vi "Utils - Convert1Dto2DImage.vi"(8 "error in (no error)":errorcluster, 9 "1DImageData In":u8[](array[numeric])) -> (0 "error out":errorcluster, 1 "1DImageData Out":u8[](array[numeric]), 2 "ImageData2D":u8[][](array[numeric]))   [LabVIEW 2015]
doc: "Convert 1d U8 Image array to LabVIEW image. This VI supports only Mono8 image format."
uses:
  xiImageManager/xiImageMng - State.ctl
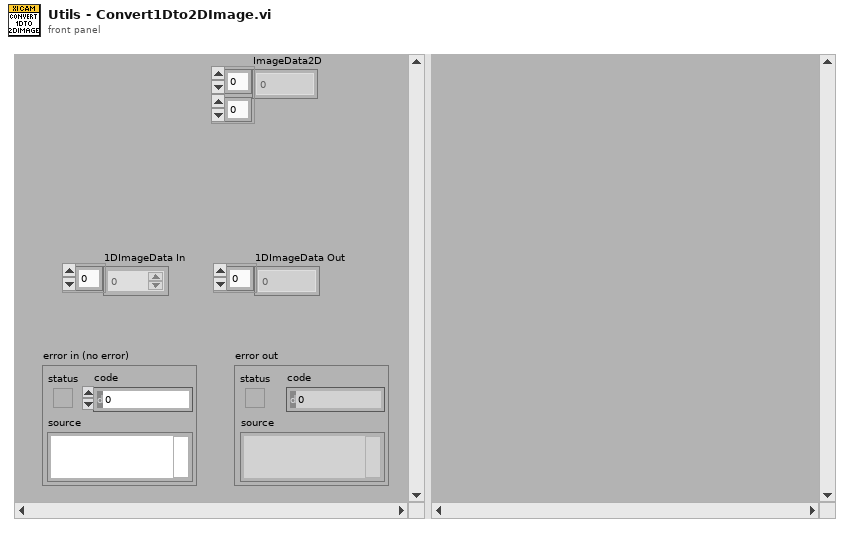
[diagram p1: front panel]
types:
  T1 = typedef "xiImageMng - State.ctl" = enum16{"Init", "GetProperties", "SetProperties"}
  T2 = typedef "xiImageMng - Attributes.ctl" = cluster{"WIDTH":i32, "HEIGHT":i32, "IMG_FORMAT":T3}
  T3 = typedef "IMG_DATA_FORMAT.ctl" = enum16{"MONO8", "MONO16", "RGB24", "RGB32", "RGBPLANAR", "RAW8", "RAW16"}
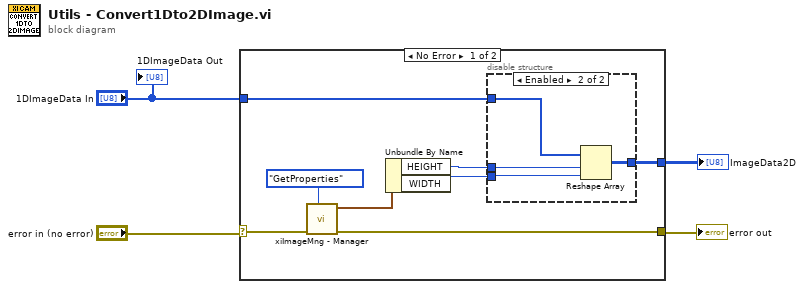
[diagram p0: block diagram]
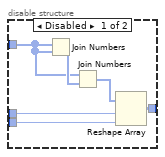
[diagram p2: hidden frame]
diagram:
  n1 = case shown="No Error" "error in (no error)" {
    selector: "error in (no error)" -> [w6 w23]
    tunnel: [w5 w23] -> w3
    tunnel: "1DImageData In" -> [w12 _]
    tunnel: [w7 _] -> w1
    frame No Error {
      n2 = call "xiImageMng - Manager.vi"("State"=xiImageMng_-_State."GetProperties", "error in (no error)"=w6) -> ("error out"=w5:errorcluster, "Properties Out"=w11:T2)  [unwired: 8 in]
      n3 = Unbundle By Name(w11) -> ("HEIGHT"=w9:i32, "WIDTH"=w8:i32)
      n4 = disable-structure shown="Enabled" {
        disable-tunnel: w12 -> [w16 w19]
        disable-tunnel: w9 -> [w15 w21]
        disable-tunnel: w8 -> [w14 w20]
        disable-tunnel: [w13 w22] -> w7
        frame Disabled {
          n5 = Join Numbers(hi=w16, lo=w16) -> ((hi.lo)=w17:u16[])
          n6 = Join Numbers(hi=w16, lo=w17) -> ((hi.lo)=w18:u32[])
          n7 = Reshape Array(w18, w15, w14) -> (w13:u32[][])
        }
        frame Enabled {
          n8 = Reshape Array(w19, w21, w20) -> (w22:u8[][])
        }
      }
    }
    frame Error {
    }
  }
  "error out" <- w3
  "ImageData2D" <- w1
  "1DImageData Out" <- "1DImageData In"
